vi "Open_Remote_Vi.vi"(8 "error in":errorcluster, 9 "Run Minimised?":bool[](array[boolean]), 10 "Remote IP":string, 11 "Vi Path":path[](array[path])) -> (0 "error out":errorcluster)   [LabVIEW 2022 SP3]
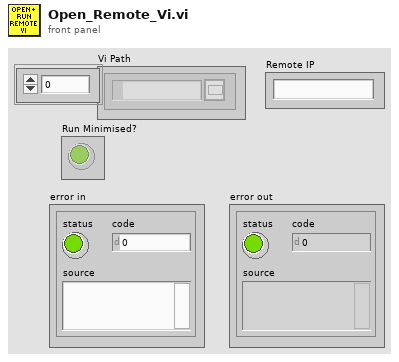
[diagram p1: front panel]
types:
  T1 = enum32{"Invalid", "Standard", "Closed", "Hidden", "Minimized", "Maximized"}
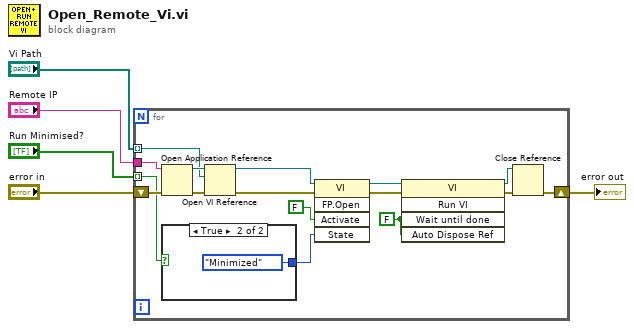
[diagram p0: block diagram]
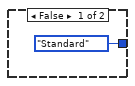
[diagram p2: hidden frame]
diagram:
  n1 = for {
    tunnel: "Vi Path" -> [w15] mode=indexing
    shift-right: [w9] -> w4
    shift-left: "error in" -> [w8]
    tunnel: "Remote IP" -> [w7]
    tunnel: "Run Minimised?" -> [w6] mode=indexing
    w18 = FALSE ("Wait Until Done")
    n2 = Open Application Reference(8:w8, 11:w7) -> (0:w12:errorcluster, 3:w16:refnum<vi>)  [unwired: 2 in]
    n3 = case shown="True" w6 {
      tunnel: [T1."Standard" ("State") T1."Minimized" ("State")] -> w19
      frame False {
      }
      frame True {
      }
    }
    n4 = Open VI Reference(application reference (local)=w16, vi path=w15, error in (no error)=w12) -> (vi reference=w10:refnum<vi>, error out=w11:errorcluster)  [unwired: 3 in]
    n5 = invoke class="VI" method="FP.Open"(reference=w10, error in=w11, "Activate"=FALSE ("Activate?"), "State"=w19) -> (reference out=w21:refnum<vi>, error out=w17:errorcluster)  [unwired: 1 in, 3 out]
    n6 = invoke class="VI" method="Run VI"(reference=w21, error in=w17, "Wait until done"=w18, "Auto Dispose Ref"=w18) -> (reference out=w14:refnum<vi>, error out=w13:errorcluster)  [unwired: 1 in, 3 out]
    n7 = Close Reference(reference=w14, error in (no error)=w13) -> (error out=w9:errorcluster)
  }
  "error out" <- w4
